vi "输入数据解析.vi"(0 "单个参数补充":dbl, 1 "从板号":dbl=1.0, 2 "主板二维码":string="BNET01", 3 "从板二维码":string="BNET01", 5 "主板引用":refnum<vi>, 7 "从板引用":refnum<vi>, 9 "主板选项":string="三级故障阀值", 11 "枚举":enum16{"主板", "从板"}(ring), 12 "快换":bool caption="快换写入") -> (4 "输出数组":dbl[][](array[numeric]), 6 "数组长度":dbl[](array[numeric]), 8 "循环次数":i32, 10 "命令":u32, 14 "名称":string[](array[string]), 15 "命令序号":u32[](array[numeric]))   [LabVIEW 2013] (continued)
          n2890 = Build Array(w7237) -> (w7236:dbl[][])
          n2891 = Build Array("一级故障阀值") -> (w7227:string[])
        }
        frame "充电电流过高(2)" {
          n2892 = Unbundle By Name(w7462) -> ("一级故障 2"=w7463:refnum<vi>)
          n2893 = property class="Clust (严格)"(reference=w7463) -> ("Value"=w7461:T4)  [unwired: 1 in, 2 out]
          n2894 = for {
            N: 17 -> [_]
            tunnel: w7461 -> [w7473]
            shift-right: [w7470] -> w7467
            shift-left: dbl[] [] -> [w7471]
            i -> [w7474]
            n2895 = case shown="13" w7474 {
              tunnel: w7473 -> [w7475 w7486 w7497 w7507 w7517 w7527 w7539 w7551 w7563 w7575 w7587 w7599 w7613 w7634 w7646 w7655 w7664]
              tunnel: [w7476 w7487 w7498 w7508 w7518 w7529 w7541 w7553 w7565 w7577 w7589 w7600 w7622 w7637 w7645 w7654 w7666] -> w7472
              frame 0, Default {
                # "总电压过高"
                n2896 = disable-structure shown="启用" {
                  disable-tunnel: [w7482 w7485] -> w7478
                  disable-tunnel: [w7481 w7485] -> w7477
                  disable-tunnel: w7475 -> [w7480 _]
                  frame Disabled {
                    n2897 = Unbundle By Name(w7480) -> ("总电压过高"=w7479:dbl)
                    n2898 = call "输入分辨率计算-EV05.vi"("1字节?"=FALSE, "数值"=w7479, "分辨率"=0.1) -> ("低字节"=w7482:dbl, "高字节1"=w7481:dbl)  [unwired: 2 in, 5 out]
                  }
                  frame Enabled {
                    w7485 = 255 ("高字节1")
                  }
                }
                n2899 = Build Array(w7477, w7478) -> (w7476:i32[])
              }
              frame 1 {
                # "总电压过低"
                n2900 = disable-structure shown="启用" {
                  disable-tunnel: [w7493 w7496] -> w7489
                  disable-tunnel: [w7492 w7496] -> w7488
                  disable-tunnel: w7486 -> [w7491 _]
                  frame Disabled {
                    n2901 = Unbundle By Name(w7491) -> ("总电压过低"=w7490:dbl)
                    n2902 = call "输入分辨率计算-EV05.vi"("1字节?"=FALSE, "数值"=w7490, "分辨率"=0.1) -> ("低字节"=w7493:dbl, "高字节1"=w7492:dbl)  [unwired: 2 in, 5 out]
                  }
                  frame Enabled {
                    w7496 = 255 ("高字节1")
                  }
                }
                n2903 = Build Array(w7488, w7489) -> (w7487:i32[])
              }
              frame 2 {
                # "温度过高"
                n2904 = disable-structure shown="启用" {
                  disable-tunnel: [w7503 255 ("高字节1")] -> w7499
                  disable-tunnel: w7497 -> [w7501 _]
                  frame Disabled {
                    n2905 = Unbundle By Name(w7501) -> ("温度过高"=w7500:dbl)
                    n2906 = call "输入分辨率计算-EV05.vi"("1字节?"=TRUE, "数值"=w7500, "偏移量"=-40.0, "分辨率"=1.0) -> ("高字节1"=w7503:dbl)  [unwired: 1 in, 6 out]
                  }
                  frame Enabled {
                  }
                }
                n2907 = Build Array(w7499) -> (w7498:i32[])
              }
              frame 3 {
                # "温度过低"
                n2908 = disable-structure shown="启用" {
                  disable-tunnel: [w7513 255 ("高字节1")] -> w7509
                  disable-tunnel: w7507 -> [w7511 _]
                  frame Disabled {
                    n2909 = Unbundle By Name(w7511) -> ("温度过低"=w7510:dbl)
                    n2910 = call "输入分辨率计算-EV05.vi"("1字节?"=TRUE, "数值"=w7510, "偏移量"=-40.0, "分辨率"=1.0) -> ("高字节1"=w7513:dbl)  [unwired: 1 in, 6 out]
                  }
                  frame Enabled {
                  }
                }
                n2911 = Build Array(w7509) -> (w7508:i32[])
              }
              frame 4 {
                # "整组温度不均衡"
                n2912 = disable-structure shown="启用" {
                  disable-tunnel: [w7523 255 ("高字节1")] -> w7519
                  disable-tunnel: w7517 -> [w7521 _]
                  frame Disabled {
                    n2913 = Unbundle By Name(w7521) -> ("整组温度不均衡"=w7520:dbl)
                    n2914 = call "输入分辨率计算-EV05.vi"("1字节?"=TRUE, "数值"=w7520, "偏移量"=0.0, "分辨率"=1.0) -> ("高字节1"=w7523:dbl)  [unwired: 1 in, 6 out]
                  }
                  frame Enabled {
                  }
                }
                n2915 = Build Array(w7519) -> (w7518:i32[])
              }
              frame 5 {
                # "单组电压不均衡"
                n2916 = disable-structure shown="启用" {
                  disable-tunnel: [w7535 w7538] -> w7530
                  disable-tunnel: [w7533 w7538] -> w7528
                  disable-tunnel: w7527 -> [w7532 _]
                  frame Disabled {
                    n2917 = Unbundle By Name(w7532) -> ("单组电压不均衡"=w7531:dbl)
                    n2918 = call "输入分辨率计算-EV05.vi"("1字节?"=FALSE, "数值"=w7531, "偏移量"=0.0, "分辨率"=0.001) -> ("低字节"=w7533:dbl, "高字节1"=w7535:dbl)  [unwired: 1 in, 5 out]
                  }
                  frame Enabled {
                    w7538 = 255 ("高字节1")
                  }
                }
                n2919 = Build Array(w7530, w7528) -> (w7529:i32[])
              }
              frame 6 {
                # "整组电压不均衡"
                n2920 = disable-structure shown="启用" {
                  disable-tunnel: [w7547 w7550] -> w7542
                  disable-tunnel: [w7545 w7550] -> w7540
                  disable-tunnel: w7539 -> [w7544 _]
                  frame Disabled {
                    n2921 = Unbundle By Name(w7544) -> ("整组电压不均衡"=w7543:dbl)
                    n2922 = call "输入分辨率计算-EV05.vi"("1字节?"=FALSE, "数值"=w7543, "偏移量"=0.0, "分辨率"=0.001) -> ("低字节"=w7545:dbl, "高字节1"=w7547:dbl)  [unwired: 1 in, 5 out]
                  }
                  frame Enabled {
                    w7550 = 255 ("高字节1")
                  }
                }
                n2923 = Build Array(w7542, w7540) -> (w7541:i32[])
              }
              frame 7 {
                # "单体电压过高"
                n2924 = disable-structure shown="启用" {
                  disable-tunnel: [w7559 w7562] -> w7554
                  disable-tunnel: [w7557 w7562] -> w7552
                  disable-tunnel: w7551 -> [w7556 _]
                  frame Disabled {
                    n2925 = Unbundle By Name(w7556) -> ("单体电压过高"=w7555:dbl)
                    n2926 = call "输入分辨率计算-EV05.vi"("1字节?"=FALSE, "数值"=w7555, "偏移量"=0.0, "分辨率"=0.001) -> ("低字节"=w7557:dbl, "高字节1"=w7559:dbl)  [unwired: 1 in, 5 out]
                  }
                  frame Enabled {
                    w7562 = 255 ("高字节1")
                  }
                }
                n2927 = Build Array(w7554, w7552) -> (w7553:i32[])
              }
              frame 8 {
                # "单体电压过低"
                n2928 = disable-structure shown="启用" {
                  disable-tunnel: [w7571 w7574] -> w7566
                  disable-tunnel: [w7569 w7574] -> w7564
                  disable-tunnel: w7563 -> [w7568 _]
                  frame Disabled {
                    n2929 = Unbundle By Name(w7568) -> ("单体电压过低"=w7567:dbl)
                    n2930 = call "输入分辨率计算-EV05.vi"("1字节?"=FALSE, "数值"=w7567, "偏移量"=0.0, "分辨率"=0.001) -> ("低字节"=w7569:dbl, "高字节1"=w7571:dbl)  [unwired: 1 in, 5 out]
                  }
                  frame Enabled {
                    w7574 = 255 ("高字节1")
                  }
                }
                n2931 = Build Array(w7566, w7564) -> (w7565:i32[])
              }
              frame 9 {
                # "充电电流过高"
                n2932 = disable-structure shown="启用" {
                  disable-tunnel: [w7583 w7586] -> w7578
                  disable-tunnel: [w7581 w7586] -> w7576
                  disable-tunnel: w7575 -> [w7580 _]
                  frame Enabled {
                    n2933 = Unbundle By Name(w7580) -> ("充电电流过高"=w7579:dbl)
                    n2934 = call "输入分辨率计算-EV05.vi"("1字节?"=FALSE, "数值"=w7579, "偏移量"=0.0, "分辨率"=0.1) -> ("低字节"=w7581:dbl, "高字节1"=w7583:dbl)  [unwired: 1 in, 5 out]
                  }
                  frame Disabled {
                    w7586 = 255 ("高字节1")
                  }
                }
                n2935 = Build Array(w7578, w7576) -> (w7577:dbl[])
              }
              frame 10 {
                # "放电电流过高"
                n2936 = disable-structure shown="启用" {
                  disable-tunnel: [w7595 w7598] -> w7590
                  disable-tunnel: [w7593 w7598] -> w7588
                  disable-tunnel: w7587 -> [w7592 _]
                  frame Disabled {
                    n2937 = Unbundle By Name(w7592) -> ("放电电流过高"=w7591:dbl)
                    n2938 = call "输入分辨率计算-EV05.vi"("1字节?"=FALSE, "数值"=w7591, "偏移量"=-3000.0, "分辨率"=0.1) -> ("低字节"=w7593:dbl, "高字节1"=w7595:dbl)  [unwired: 1 in, 5 out]
                  }
                  frame Enabled {
                    w7598 = 255 ("高字节1")
                  }
                }
                n2939 = Build Array(w7590, w7588) -> (w7589:i32[])
              }
              frame 11 {
                # "单组温度不均衡"
                n2940 = disable-structure shown="启用" {
                  disable-tunnel: [w7605 255 ("高字节1")] -> w7601
                  disable-tunnel: w7599 -> [w7603 _]
                  frame Disabled {
                    n2941 = Unbundle By Name(w7603) -> ("单组温度不均衡"=w7602:dbl)
                    n2942 = call "输入分辨率计算-EV05.vi"("1字节?"=TRUE, "数值"=w7602, "偏移量"=0.0, "分辨率"=1.0) -> ("高字节1"=w7605:dbl)  [unwired: 1 in, 6 out]
                  }
                  frame Enabled {
                  }
                }
                n2943 = Build Array(w7601) -> (w7600:i32[])
              }
              frame 12 {
                # "SOC过高"
                n2944 = Unbundle By Name(w7613) -> ("SOC过高"=w7612:dbl)
                n2945 = call "输入分辨率计算-EV05.vi"("1字节?"=FALSE, "数值"=w7612, "偏移量"=0.0, "分辨率"=0.1) -> ("低字节"=w7614:dbl, "高字节1"=w7615:dbl)  [unwired: 1 in, 5 out]
                n2946 = call "二进制解析-8.6.vi"("索引"=4, "数值"=w7615) -> ("低位子数组"=w7618:i32[])  [unwired: 3 out]
                n2947 = call "二进制解析-8.6.vi"("索引"=4, "数值"=w7614) -> ("低位子数组"=w7610:i32[], "高位子数组"=w7617:i32[])  [unwired: 2 out]
                n2948 = Insert Into Array(array=w7618, new element=w7617) -> (w7616:i32[])  [unwired: 1 in]
                n2949 = call "数值二进制转十进制-8.6.vi"("子数组"=w7616) -> ("十进制数值"=w7611:i32)  [unwired: 4 out]
                n2950 = disable-structure shown="启用" {
                  disable-tunnel: w7611 -> [w7626 _]
                  disable-tunnel: [w7626 255 ("高字节1")] -> w7609
                  disable-tunnel: [w7625 i32[] [] ("低位子数组 27")] -> _
                  disable-tunnel: w7610 -> [w7625 _]
                  frame Disabled {
                  }
                  frame Enabled {
                  }
                }
                n2951 = Build Array(w7609, w7609) -> (w7622:i32[])
              }
              frame 13 {
                # "SOC过低"
                n2952 = Unbundle By Name(w7634) -> ("SOC过低"=w7633:dbl)
                n2953 = call "输入分辨率计算-EV05.vi"("1字节?"=FALSE, "数值"=w7633, "偏移量"=0.0, "分辨率"=0.1) -> ("低字节"=w7631:dbl, "高字节1"=w7632:dbl)  [unwired: 1 in, 5 out]
                n2954 = call "二进制解析-8.6.vi"("索引"=4, "数值"=w7632) -> ("低位子数组"=w7630:i32[])  [unwired: 3 out]
                n2955 = disable-structure shown="启用" {
                  disable-tunnel: w7631 -> [w7641 _]
                  disable-tunnel: [w7641 255 ("高字节1")] -> w7629
                  disable-tunnel: w7630 -> [w7640 _]
                  disable-tunnel: [w7640 i32[] [] ("低位子数组")] -> _
                  frame Disabled {
                    (unwired) i32[] [] ("低位子数组 4")
                  }
                  frame Enabled {
                  }
                }
                n2956 = Build Array(w7629, w7629) -> (w7637:i32[])
              }
              frame 14 {
                # "内阻过大"
                n2957 = disable-structure shown="启用" {
                  disable-tunnel: w7646 -> [w7651 _]
                  disable-tunnel: [w7647 255 ("高字节1")] -> w7644
                  frame Disabled {
                    n2958 = Unbundle By Name(w7651) -> ("内阻过大"=w7650:dbl)
                    n2959 = call "输入分辨率计算-EV05.vi"("1字节?"=TRUE, "数值"=w7650, "分辨率"=0.1) -> ("高字节1"=w7647:dbl)  [unwired: 2 in, 6 out]
                  }
                  frame Enabled {
                  }
                }
                n2960 = Build Array(w7644) -> (w7645:i32[])
              }
              frame 15 {
                # "极柱温度过高"
                n2961 = disable-structure shown="启用" {
                  disable-tunnel: w7655 -> [w7661 _]
                  disable-tunnel: [w7657 255 ("高字节1")] -> w7653
                  frame Disabled {
                    n2962 = Unbundle By Name(w7661) -> ("极柱温度过高"=w7660:dbl)
                    n2963 = call "输入分辨率计算-EV05.vi"("1字节?"=TRUE, "数值"=w7660, "偏移量"=-40.0, "分辨率"=1.0) -> ("高字节1"=w7657:dbl)  [unwired: 1 in, 6 out]
                  }
                  frame Enabled {
                  }
                }
                n2964 = Build Array(w7653) -> (w7654:i32[])
              }
              frame 16 {
                # "SOH过低"
                n2965 = disable-structure shown="启用" {
                  disable-tunnel: [w7678 w7686] -> w7665
                  disable-tunnel: w7664 -> [w7675 _]
                  disable-tunnel: [w7667 w7686] -> w7663
                  frame Disabled {
                    n2966 = Unbundle By Name(w7675) -> ("SOH过低"=w7674:dbl)
                    n2967 = call "输入分辨率计算-EV05.vi"("1字节?"=FALSE, "数值"=w7674, "偏移量"=0.0, "分辨率"=0.1) -> ("低字节"=w7676:dbl, "高字节1"=w7677:dbl)  [unwired: 1 in, 5 out]
                    n2968 = call "二进制解析-8.6.vi"("索引"=4, "数值"=w7677) -> ("低位子数组"=w7680:i32[])  [unwired: 3 out]
                    n2969 = call "二进制解析-8.6.vi"("索引"=4, "数值"=w7676) -> ("低位子数组"=w7669:i32[], "高位子数组"=w7679:i32[])  [unwired: 2 out]
                    n2970 = call "二进制解析-8.6.vi"("索引"=4, "数值"=0) -> ("低位子数组"=w7670:i32[])  [unwired: 3 out]
                    n2971 = Insert Into Array(array=w7680, new element=w7679) -> (w7673:i32[])  [unwired: 1 in]
                    n2972 = Insert Into Array(array=w7669, new element=w7670) -> (w7668:i32[])  [unwired: 1 in]
                    n2973 = call "数值二进制转十进制-8.6.vi"("子数组"=w7673) -> ("十进制数值"=w7678:i32)  [unwired: 4 out]
                    n2974 = call "数值二进制转十进制-8.6.vi"("子数组"=w7668) -> ("十进制数值"=w7667:i32)  [unwired: 4 out]
                  }
                  frame Enabled {
                    w7686 = 255 ("高字节1")
                  }
                }
                n2975 = Build Array(w7665, w7663) -> (w7666:i32[])
              }
            }
            n2976 = Insert Into Array(array=w7471, new element=w7472) -> (w7470:dbl[])  [unwired: 1 in]
          }
          n2977 = Build Array(w7467) -> (w7466:dbl[][])
          n2978 = Build Array("二级故障阀值") -> (w7457:string[])
        }
        frame "充电电流过高(3)" {
          n2979 = Unbundle By Name(w7692) -> ("一级故障 3"=w7693:refnum<vi>)
          n2980 = property class="Clust (严格)"(reference=w7693) -> ("Value"=w7691:T4)  [unwired: 1 in, 2 out]
          n2981 = for {
            N: 17 -> [_]
            tunnel: w7691 -> [w7703]
            shift-right: [w7700] -> w7697
            shift-left: dbl[] [] -> [w7701]
            i -> [w7704]
            n2982 = case shown="13" w7704 {
              tunnel: w7703 -> [w7705 w7716 w7727 w7737 w7747 w7757 w7769 w7781 w7793 w7805 w7817 w7829 w7843 w7864 w7876 w7885 w7894]
              tunnel: [w7706 w7717 w7728 w7738 w7748 w7759 w7771 w7783 w7795 w7807 w7819 w7830 w7852 w7867 w7875 w7884 w7896] -> w7702
              frame 0, Default {
                # "总电压过高"
                n2983 = disable-structure shown="启用" {
                  disable-tunnel: [w7712 w7715] -> w7708
                  disable-tunnel: [w7711 w7715] -> w7707
                  disable-tunnel: w7705 -> [w7710 _]
                  frame Disabled {
                    n2984 = Unbundle By Name(w7710) -> ("总电压过高"=w7709:dbl)
                    n2985 = call "输入分辨率计算-EV05.vi"("1字节?"=FALSE, "数值"=w7709, "分辨率"=0.1) -> ("低字节"=w7712:dbl, "高字节1"=w7711:dbl)  [unwired: 2 in, 5 out]
                  }
                  frame Enabled {
                    w7715 = 255 ("高字节1")
                  }
                }
                n2986 = Build Array(w7707, w7708) -> (w7706:i32[])
              }
              frame 1 {
                # "总电压过低"
                n2987 = disable-structure shown="启用" {
                  disable-tunnel: [w7723 w7726] -> w7719
                  disable-tunnel: [w7722 w7726] -> w7718
                  disable-tunnel: w7716 -> [w7721 _]
                  frame Disabled {
                    n2988 = Unbundle By Name(w7721) -> ("总电压过低"=w7720:dbl)
                    n2989 = call "输入分辨率计算-EV05.vi"("1字节?"=FALSE, "数值"=w7720, "分辨率"=0.1) -> ("低字节"=w7723:dbl, "高字节1"=w7722:dbl)  [unwired: 2 in, 5 out]
                  }
                  frame Enabled {
                    w7726 = 255 ("高字节1")
                  }
                }
                n2990 = Build Array(w7718, w7719) -> (w7717:i32[])
              }
              frame 2 {
                # "温度过高"
                n2991 = disable-structure shown="启用" {
                  disable-tunnel: [w7733 255 ("高字节1")] -> w7729
                  disable-tunnel: w7727 -> [w7731 _]
                  frame Disabled {
                    n2992 = Unbundle By Name(w7731) -> ("温度过高"=w7730:dbl)
                    n2993 = call "输入分辨率计算-EV05.vi"("1字节?"=TRUE, "数值"=w7730, "偏移量"=-40.0, "分辨率"=1.0) -> ("高字节1"=w7733:dbl)  [unwired: 1 in, 6 out]
                  }
                  frame Enabled {
                  }
                }
                n2994 = Build Array(w7729) -> (w7728:i32[])
              }
              frame 3 {
                # "温度过低"
                n2995 = disable-structure shown="启用" {
                  disable-tunnel: [w7743 255 ("高字节1")] -> w7739
                  disable-tunnel: w7737 -> [w7741 _]
                  frame Disabled {
                    n2996 = Unbundle By Name(w7741) -> ("温度过低"=w7740:dbl)
                    n2997 = call "输入分辨率计算-EV05.vi"("1字节?"=TRUE, "数值"=w7740, "偏移量"=-40.0, "分辨率"=1.0) -> ("高字节1"=w7743:dbl)  [unwired: 1 in, 6 out]
                  }
                  frame Enabled {
                  }
                }
                n2998 = Build Array(w7739) -> (w7738:i32[])
              }
              frame 4 {
                # "整组温度不均衡"
                n2999 = disable-structure shown="启用" {
                  disable-tunnel: [w7753 255 ("高字节1")] -> w7749
                  disable-tunnel: w7747 -> [w7751 _]
                  frame Disabled {
                    n3000 = Unbundle By Name(w7751) -> ("整组温度不均衡"=w7750:dbl)
                    n3001 = call "输入分辨率计算-EV05.vi"("1字节?"=TRUE, "数值"=w7750, "偏移量"=0.0, "分辨率"=1.0) -> ("高字节1"=w7753:dbl)  [unwired: 1 in, 6 out]
                  }
                  frame Enabled {
                  }
                }
                n3002 = Build Array(w7749) -> (w7748:i32[])
              }
              frame 5 {
                # "单组电压不均衡"
                n3003 = disable-structure shown="启用" {
                  disable-tunnel: [w7765 w7768] -> w7760
                  disable-tunnel: [w7763 w7768] -> w7758
                  disable-tunnel: w7757 -> [w7762 _]
                  frame Disabled {
                    n3004 = Unbundle By Name(w7762) -> ("单组电压不均衡"=w7761:dbl)
                    n3005 = call "输入分辨率计算-EV05.vi"("1字节?"=FALSE, "数值"=w7761, "偏移量"=0.0, "分辨率"=0.001) -> ("低字节"=w7763:dbl, "高字节1"=w7765:dbl)  [unwired: 1 in, 5 out]
                  }
                  frame Enabled {
                    w7768 = 255 ("高字节1")
                  }
                }
                n3006 = Build Array(w7760, w7758) -> (w7759:i32[])
              }
              frame 6 {
                # "整组电压不均衡"
                n3007 = disable-structure shown="启用" {
                  disable-tunnel: [w7777 w7780] -> w7772
                  disable-tunnel: [w7775 w7780] -> w7770
                  disable-tunnel: w7769 -> [w7774 _]
                  frame Disabled {
                    n3008 = Unbundle By Name(w7774) -> ("整组电压不均衡"=w7773:dbl)
                    n3009 = call "输入分辨率计算-EV05.vi"("1字节?"=FALSE, "数值"=w7773, "偏移量"=0.0, "分辨率"=0.001) -> ("低字节"=w7775:dbl, "高字节1"=w7777:dbl)  [unwired: 1 in, 5 out]
                  }
                  frame Enabled {
                    w7780 = 255 ("高字节1")
                  }
                }
                n3010 = Build Array(w7772, w7770) -> (w7771:i32[])
              }
              frame 7 {
                # "单体电压过高"
                n3011 = disable-structure shown="启用" {
                  disable-tunnel: [w7789 w7792] -> w7784
                  disable-tunnel: [w7787 w7792] -> w7782
                  disable-tunnel: w7781 -> [w7786 _]
                  frame Disabled {
                    n3012 = Unbundle By Name(w7786) -> ("单体电压过高"=w7785:dbl)
                    n3013 = call "输入分辨率计算-EV05.vi"("1字节?"=FALSE, "数值"=w7785, "偏移量"=0.0, "分辨率"=0.001) -> ("低字节"=w7787:dbl, "高字节1"=w7789:dbl)  [unwired: 1 in, 5 out]
                  }
                  frame Enabled {
                    w7792 = 255 ("高字节1")
                  }
                }
                n3014 = Build Array(w7784, w7782) -> (w7783:i32[])
              }
              frame 8 {
                # "单体电压过低"
                n3015 = disable-structure shown="启用" {
                  disable-tunnel: [w7801 w7804] -> w7796
                  disable-tunnel: [w7799 w7804] -> w7794
                  disable-tunnel: w7793 -> [w7798 _]
                  frame Disabled {
                    n3016 = Unbundle By Name(w7798) -> ("单体电压过低"=w7797:dbl)
                    n3017 = call "输入分辨率计算-EV05.vi"("1字节?"=FALSE, "数值"=w7797, "偏移量"=0.0, "分辨率"=0.001) -> ("低字节"=w7799:dbl, "高字节1"=w7801:dbl)  [unwired: 1 in, 5 out]
                  }
                  frame Enabled {
                    w7804 = 255 ("高字节1")
                  }
                }
                n3018 = Build Array(w7796, w7794) -> (w7795:i32[])
              }
              frame 9 {
                # "充电电流过高"
                n3019 = disable-structure shown="启用" {
                  disable-tunnel: [w7813 w7816] -> w7808
                  disable-tunnel: [w7811 w7816] -> w7806
                  disable-tunnel: w7805 -> [w7810 _]
                  frame Enabled {
                    n3020 = Unbundle By Name(w7810) -> ("充电电流过高"=w7809:dbl)
                    n3021 = call "输入分辨率计算-EV05.vi"("1字节?"=FALSE, "数值"=w7809, "偏移量"=0.0, "分辨率"=0.1) -> ("低字节"=w7811:dbl, "高字节1"=w7813:dbl)  [unwired: 1 in, 5 out]
                  }
                  frame Disabled {
                    w7816 = 255 ("高字节1")
                  }
                }
                n3022 = Build Array(w7808, w7806) -> (w7807:dbl[])
              }
              frame 10 {
                # "放电电流过高"
                n3023 = disable-structure shown="启用" {
                  disable-tunnel: [w7825 w7828] -> w7820
                  disable-tunnel: [w7823 w7828] -> w7818
                  disable-tunnel: w7817 -> [w7822 _]
                  frame Disabled {
                    n3024 = Unbundle By Name(w7822) -> ("放电电流过高"=w7821:dbl)
                    n3025 = call "输入分辨率计算-EV05.vi"("1字节?"=FALSE, "数值"=w7821, "偏移量"=-3000.0, "分辨率"=0.1) -> ("低字节"=w7823:dbl, "高字节1"=w7825:dbl)  [unwired: 1 in, 5 out]
                  }
                  frame Enabled {
                    w7828 = 255 ("高字节1")
                  }
                }
                n3026 = Build Array(w7820, w7818) -> (w7819:i32[])
              }
              frame 11 {
                # "单组温度不均衡"
                n3027 = disable-structure shown="启用" {
                  disable-tunnel: [w7835 255 ("高字节1")] -> w7831
                  disable-tunnel: w7829 -> [w7833 _]
                  frame Disabled {
                    n3028 = Unbundle By Name(w7833) -> ("单组温度不均衡"=w7832:dbl)
                    n3029 = call "输入分辨率计算-EV05.vi"("1字节?"=TRUE, "数值"=w7832, "偏移量"=0.0, "分辨率"=1.0) -> ("高字节1"=w7835:dbl)  [unwired: 1 in, 6 out]
                  }
                  frame Enabled {
                  }
                }
                n3030 = Build Array(w7831) -> (w7830:i32[])
              }
              frame 12 {
                # "SOC过高"
                n3031 = Unbundle By Name(w7843) -> ("SOC过高"=w7842:dbl)
                n3032 = call "输入分辨率计算-EV05.vi"("1字节?"=FALSE, "数值"=w7842, "偏移量"=0.0, "分辨率"=0.1) -> ("低字节"=w7844:dbl, "高字节1"=w7845:dbl)  [unwired: 1 in, 5 out]
                n3033 = call "二进制解析-8.6.vi"("索引"=4, "数值"=w7845) -> ("低位子数组"=w7848:i32[])  [unwired: 3 out]
                n3034 = call "二进制解析-8.6.vi"("索引"=4, "数值"=w7844) -> ("低位子数组"=w7840:i32[], "高位子数组"=w7847:i32[])  [unwired: 2 out]
                n3035 = Insert Into Array(array=w7848, new element=w7847) -> (w7846:i32[])  [unwired: 1 in]
                n3036 = call "数值二进制转十进制-8.6.vi"("子数组"=w7846) -> ("十进制数值"=w7841:i32)  [unwired: 4 out]
                n3037 = disable-structure shown="启用" {
                  disable-tunnel: w7841 -> [w7856 _]
                  disable-tunnel: [w7856 255 ("高字节1")] -> w7839
                  disable-tunnel: [w7855 i32[] [] ("低位子数组 27")] -> _
                  disable-tunnel: w7840 -> [w7855 _]
                  frame Disabled {
                  }
                  frame Enabled {
                  }
                }
                n3038 = Build Array(w7839, w7839) -> (w7852:i32[])
              }
              frame 13 {
                # "SOC过低"
                n3039 = Unbundle By Name(w7864) -> ("SOC过低"=w7863:dbl)
                n3040 = call "输入分辨率计算-EV05.vi"("1字节?"=FALSE, "数值"=w7863, "偏移量"=0.0, "分辨率"=0.1) -> ("低字节"=w7861:dbl, "高字节1"=w7862:dbl)  [unwired: 1 in, 5 out]
                n3041 = call "二进制解析-8.6.vi"("索引"=4, "数值"=w7862) -> ("低位子数组"=w7860:i32[])  [unwired: 3 out]
                n3042 = disable-structure shown="启用" {
                  disable-tunnel: w7861 -> [w7871 _]
                  disable-tunnel: [w7871 255 ("高字节1")] -> w7859
                  disable-tunnel: w7860 -> [w7870 _]
                  disable-tunnel: [w7870 i32[] [] ("低位子数组")] -> _
                  frame Disabled {
                    (unwired) i32[] [] ("低位子数组 4")
                  }
                  frame Enabled {
                  }
                }
                n3043 = Build Array(w7859, w7859) -> (w7867:i32[])
              }
              frame 14 {
                # "内阻过大"
                n3044 = disable-structure shown="启用" {
                  disable-tunnel: w7876 -> [w7881 _]
                  disable-tunnel: [w7877 255 ("高字节1")] -> w7874
                  frame Disabled {
                    n3045 = Unbundle By Name(w7881) -> ("内阻过大"=w7880:dbl)
                    n3046 = call "输入分辨率计算-EV05.vi"("1字节?"=TRUE, "数值"=w7880, "分辨率"=0.1) -> ("高字节1"=w7877:dbl)  [unwired: 2 in, 6 out]
                  }
                  frame Enabled {
                  }
                }
                n3047 = Build Array(w7874) -> (w7875:i32[])
              }
              frame 15 {
                # "极柱温度过高"
                n3048 = disable-structure shown="启用" {
                  disable-tunnel: w7885 -> [w7891 _]
                  disable-tunnel: [w7887 255 ("高字节1")] -> w7883
                  frame Disabled {
                    n3049 = Unbundle By Name(w7891) -> ("极柱温度过高"=w7890:dbl)
                    n3050 = call "输入分辨率计算-EV05.vi"("1字节?"=TRUE, "数值"=w7890, "偏移量"=-40.0, "分辨率"=1.0) -> ("高字节1"=w7887:dbl)  [unwired: 1 in, 6 out]
                  }
                  frame Enabled {
                  }
                }
                n3051 = Build Array(w7883) -> (w7884:i32[])
              }
              frame 16 {
                # "SOH过低"
                n3052 = disable-structure shown="启用" {
                  disable-tunnel: [w7908 w7916] -> w7895
                  disable-tunnel: w7894 -> [w7905 _]
                  disable-tunnel: [w7897 w7916] -> w7893
                  frame Disabled {
                    n3053 = Unbundle By Name(w7905) -> ("SOH过低"=w7904:dbl)
                    n3054 = call "输入分辨率计算-EV05.vi"("1字节?"=FALSE, "数值"=w7904, "偏移量"=0.0, "分辨率"=0.1) -> ("低字节"=w7906:dbl, "高字节1"=w7907:dbl)  [unwired: 1 in, 5 out]
                    n3055 = call "二进制解析-8.6.vi"("索引"=4, "数值"=w7907) -> ("低位子数组"=w7910:i32[])  [unwired: 3 out]
                    n3056 = call "二进制解析-8.6.vi"("索引"=4, "数值"=w7906) -> ("低位子数组"=w7899:i32[], "高位子数组"=w7909:i32[])  [unwired: 2 out]
                    n3057 = call "二进制解析-8.6.vi"("索引"=4, "数值"=0) -> ("低位子数组"=w7900:i32[])  [unwired: 3 out]
                    n3058 = Insert Into Array(array=w7910, new element=w7909) -> (w7903:i32[])  [unwired: 1 in]
                    n3059 = Insert Into Array(array=w7899, new element=w7900) -> (w7898:i32[])  [unwired: 1 in]
                    n3060 = call "数值二进制转十进制-8.6.vi"("子数组"=w7903) -> ("十进制数值"=w7908:i32)  [unwired: 4 out]
                    n3061 = call "数值二进制转十进制-8.6.vi"("子数组"=w7898) -> ("十进制数值"=w7897:i32)  [unwired: 4 out]
                  }
                  frame Enabled {
                    w7916 = 255 ("高字节1")
                  }
                }
                n3062 = Build Array(w7895, w7893) -> (w7896:i32[])
              }
            }
            n3063 = Insert Into Array(array=w7701, new element=w7702) -> (w7700:dbl[])  [unwired: 1 in]
          }
          n3064 = Build Array(w7697) -> (w7696:dbl[][])
          n3065 = Build Array("三级故障阀值") -> (w7687:string[])
        }
        frame "放电电流过高" {
          n3066 = Unbundle By Name(w7922) -> ("一级故障"=w7923:refnum<vi>)
          n3067 = property class="Clust (严格)"(reference=w7923) -> ("Value"=w7921:T4)  [unwired: 1 in, 2 out]
          n3068 = for {
            N: 17 -> [_]
            tunnel: w7921 -> [w7933]
            shift-right: [w7930] -> w7927
            shift-left: dbl[] [] -> [w7931]
            i -> [w7934]
            n3069 = case shown="14" w7934 {
              tunnel: w7933 -> [w7935 w7946 w7957 w7967 w7977 w7987 w7999 w8011 w8023 w8035 w8047 w8059 w8073 w8094 w8106 w8115 w8124]
              tunnel: [w7936 w7947 w7958 w7968 w7978 w7989 w8001 w8013 w8025 w8037 w8049 w8060 w8082 w8097 w8105 w8114 w8126] -> w7932
              frame 0, Default {
                # "总电压过高"
                n3070 = disable-structure shown="启用" {
                  disable-tunnel: [w7942 w7945] -> w7938
                  disable-tunnel: [w7941 w7945] -> w7937
                  disable-tunnel: w7935 -> [w7940 _]
                  frame Disabled {
                    n3071 = Unbundle By Name(w7940) -> ("总电压过高"=w7939:dbl)
                    n3072 = call "输入分辨率计算-EV05.vi"("1字节?"=FALSE, "数值"=w7939, "分辨率"=0.1) -> ("低字节"=w7942:dbl, "高字节1"=w7941:dbl)  [unwired: 2 in, 5 out]
                  }
                  frame Enabled {
                    w7945 = 255 ("高字节1")
                  }
                }
                n3073 = Build Array(w7937, w7938) -> (w7936:i32[])
              }
              frame 1 {
                # "总电压过低"
                n3074 = disable-structure shown="启用" {
                  disable-tunnel: [w7953 w7956] -> w7949
                  disable-tunnel: [w7952 w7956] -> w7948
                  disable-tunnel: w7946 -> [w7951 _]
                  frame Disabled {
                    n3075 = Unbundle By Name(w7951) -> ("总电压过低"=w7950:dbl)
                    n3076 = call "输入分辨率计算-EV05.vi"("1字节?"=FALSE, "数值"=w7950, "分辨率"=0.1) -> ("低字节"=w7953:dbl, "高字节1"=w7952:dbl)  [unwired: 2 in, 5 out]
                  }
                  frame Enabled {
                    w7956 = 255 ("高字节1")
                  }
                }
                n3077 = Build Array(w7948, w7949) -> (w7947:i32[])
              }
              frame 2 {
                # "温度过高"
                n3078 = disable-structure shown="启用" {
                  disable-tunnel: [w7963 255 ("高字节1")] -> w7959
                  disable-tunnel: w7957 -> [w7961 _]
                  frame Disabled {
                    n3079 = Unbundle By Name(w7961) -> ("温度过高"=w7960:dbl)
                    n3080 = call "输入分辨率计算-EV05.vi"("1字节?"=TRUE, "数值"=w7960, "偏移量"=-40.0, "分辨率"=1.0) -> ("高字节1"=w7963:dbl)  [unwired: 1 in, 6 out]
                  }
                  frame Enabled {
                  }
                }
                n3081 = Build Array(w7959) -> (w7958:i32[])
              }
              frame 3 {
                # "温度过低"
                n3082 = disable-structure shown="启用" {
                  disable-tunnel: [w7973 255 ("高字节1")] -> w7969
                  disable-tunnel: w7967 -> [w7971 _]
                  frame Disabled {
                    n3083 = Unbundle By Name(w7971) -> ("温度过低"=w7970:dbl)
                    n3084 = call "输入分辨率计算-EV05.vi"("1字节?"=TRUE, "数值"=w7970, "偏移量"=-40.0, "分辨率"=1.0) -> ("高字节1"=w7973:dbl)  [unwired: 1 in, 6 out]
                  }
                  frame Enabled {
                  }
                }
                n3085 = Build Array(w7969) -> (w7968:i32[])
              }
              frame 4 {
                # "整组温度不均衡"
                n3086 = disable-structure shown="启用" {
                  disable-tunnel: [w7983 255 ("高字节1")] -> w7979
                  disable-tunnel: w7977 -> [w7981 _]
                  frame Disabled {
                    n3087 = Unbundle By Name(w7981) -> ("整组温度不均衡"=w7980:dbl)
                    n3088 = call "输入分辨率计算-EV05.vi"("1字节?"=TRUE, "数值"=w7980, "偏移量"=0.0, "分辨率"=1.0) -> ("高字节1"=w7983:dbl)  [unwired: 1 in, 6 out]
                  }
                  frame Enabled {
                  }
                }
                n3089 = Build Array(w7979) -> (w7978:i32[])
              }
              frame 5 {
                # "单组电压不均衡"
                n3090 = disable-structure shown="启用" {
                  disable-tunnel: [w7995 w7998] -> w7990
                  disable-tunnel: [w7993 w7998] -> w7988
                  disable-tunnel: w7987 -> [w7992 _]
                  frame Disabled {
                    n3091 = Unbundle By Name(w7992) -> ("单组电压不均衡"=w7991:dbl)
                    n3092 = call "输入分辨率计算-EV05.vi"("1字节?"=FALSE, "数值"=w7991, "偏移量"=0.0, "分辨率"=0.001) -> ("低字节"=w7993:dbl, "高字节1"=w7995:dbl)  [unwired: 1 in, 5 out]
                  }
                  frame Enabled {
                    w7998 = 255 ("高字节1")
                  }
                }
                n3093 = Build Array(w7990, w7988) -> (w7989:i32[])
              }
              frame 6 {
                # "整组电压不均衡"
                n3094 = disable-structure shown="启用" {
                  disable-tunnel: [w8007 w8010] -> w8002
                  disable-tunnel: [w8005 w8010] -> w8000
                  disable-tunnel: w7999 -> [w8004 _]
                  frame Disabled {
                    n3095 = Unbundle By Name(w8004) -> ("整组电压不均衡"=w8003:dbl)
                    n3096 = call "输入分辨率计算-EV05.vi"("1字节?"=FALSE, "数值"=w8003, "偏移量"=0.0, "分辨率"=0.001) -> ("低字节"=w8005:dbl, "高字节1"=w8007:dbl)  [unwired: 1 in, 5 out]
                  }
                  frame Enabled {
                    w8010 = 255 ("高字节1")
                  }
                }
                n3097 = Build Array(w8002, w8000) -> (w8001:i32[])
              }
              frame 7 {
                # "单体电压过高"
                n3098 = disable-structure shown="启用" {
                  disable-tunnel: [w8019 w8022] -> w8014
                  disable-tunnel: [w8017 w8022] -> w8012
                  disable-tunnel: w8011 -> [w8016 _]
                  frame Disabled {
                    n3099 = Unbundle By Name(w8016) -> ("单体电压过高"=w8015:dbl)
                    n3100 = call "输入分辨率计算-EV05.vi"("1字节?"=FALSE, "数值"=w8015, "偏移量"=0.0, "分辨率"=0.001) -> ("低字节"=w8017:dbl, "高字节1"=w8019:dbl)  [unwired: 1 in, 5 out]
                  }
                  frame Enabled {
                    w8022 = 255 ("高字节1")
                  }
                }
                n3101 = Build Array(w8014, w8012) -> (w8013:i32[])
              }
              frame 8 {
                # "单体电压过低"
                n3102 = disable-structure shown="启用" {
                  disable-tunnel: [w8031 w8034] -> w8026
                  disable-tunnel: [w8029 w8034] -> w8024
                  disable-tunnel: w8023 -> [w8028 _]
                  frame Disabled {
                    n3103 = Unbundle By Name(w8028) -> ("单体电压过低"=w8027:dbl)
                    n3104 = call "输入分辨率计算-EV05.vi"("1字节?"=FALSE, "数值"=w8027, "偏移量"=0.0, "分辨率"=0.001) -> ("低字节"=w8029:dbl, "高字节1"=w8031:dbl)  [unwired: 1 in, 5 out]
                  }
                  frame Enabled {
                    w8034 = 255 ("高字节1")
                  }
                }
                n3105 = Build Array(w8026, w8024) -> (w8025:i32[])
              }
              frame 9 {
                # "充电电流过高"
                n3106 = disable-structure shown="启用" {
                  disable-tunnel: [w8043 w8046] -> w8038
                  disable-tunnel: [w8041 w8046] -> w8036
                  disable-tunnel: w8035 -> [w8040 _]
                  frame Disabled {
                    n3107 = Unbundle By Name(w8040) -> ("充电电流过高"=w8039:dbl)
                    n3108 = call "输入分辨率计算-EV05.vi"("1字节?"=FALSE, "数值"=w8039, "偏移量"=-3000.0, "分辨率"=0.1) -> ("低字节"=w8041:dbl, "高字节1"=w8043:dbl)  [unwired: 1 in, 5 out]
                  }
                  frame Enabled {
                    w8046 = 255 ("高字节1")
                  }
                }
                n3109 = Build Array(w8038, w8036) -> (w8037:i32[])
              }
              frame 10 {
                # "放电电流过高"
                n3110 = disable-structure shown="启用" {
                  disable-tunnel: [w8055 w8058] -> w8050
                  disable-tunnel: [w8053 w8058] -> w8048
                  disable-tunnel: w8047 -> [w8052 _]
                  frame Enabled {
                    n3111 = Unbundle By Name(w8052) -> ("放电电流过高"=w8051:dbl)
                    n3112 = call "输入分辨率计算-EV05.vi"("1字节?"=FALSE, "数值"=w8051, "偏移量"=0.0, "分辨率"=0.1) -> ("低字节"=w8053:dbl, "高字节1"=w8055:dbl)  [unwired: 1 in, 5 out]
                  }
                  frame Disabled {
                    w8058 = 255 ("高字节1")
                  }
                }
                n3113 = Build Array(w8050, w8048) -> (w8049:dbl[])
              }
              frame 11 {
                # "单组温度不均衡"
                n3114 = disable-structure shown="启用" {
                  disable-tunnel: [w8065 255 ("高字节1")] -> w8061
                  disable-tunnel: w8059 -> [w8063 _]
                  frame Disabled {
                    n3115 = Unbundle By Name(w8063) -> ("单组温度不均衡"=w8062:dbl)
                    n3116 = call "输入分辨率计算-EV05.vi"("1字节?"=TRUE, "数值"=w8062, "偏移量"=0.0, "分辨率"=1.0) -> ("高字节1"=w8065:dbl)  [unwired: 1 in, 6 out]
                  }
                  frame Enabled {
                  }
                }
                n3117 = Build Array(w8061) -> (w8060:i32[])
              }
              frame 12 {
                # "SOC过高"
                n3118 = Unbundle By Name(w8073) -> ("SOC过高"=w8072:dbl)
                n3119 = call "输入分辨率计算-EV05.vi"("1字节?"=FALSE, "数值"=w8072, "偏移量"=0.0, "分辨率"=0.1) -> ("低字节"=w8074:dbl, "高字节1"=w8075:dbl)  [unwired: 1 in, 5 out]
                n3120 = call "二进制解析-8.6.vi"("索引"=4, "数值"=w8075) -> ("低位子数组"=w8078:i32[])  [unwired: 3 out]
                n3121 = call "二进制解析-8.6.vi"("索引"=4, "数值"=w8074) -> ("低位子数组"=w8070:i32[], "高位子数组"=w8077:i32[])  [unwired: 2 out]
                n3122 = Insert Into Array(array=w8078, new element=w8077) -> (w8076:i32[])  [unwired: 1 in]
                n3123 = call "数值二进制转十进制-8.6.vi"("子数组"=w8076) -> ("十进制数值"=w8071:i32)  [unwired: 4 out]
                n3124 = disable-structure shown="启用" {
                  disable-tunnel: w8071 -> [w8086 _]
                  disable-tunnel: [w8086 255 ("高字节1")] -> w8069
                  disable-tunnel: [w8085 i32[] [] ("低位子数组 28")] -> _
                  disable-tunnel: w8070 -> [w8085 _]
                  frame Disabled {
                  }
                  frame Enabled {
                  }
                }
                n3125 = Build Array(w8069, w8069) -> (w8082:i32[])
              }
              frame 13 {
                # "SOC过低"
                n3126 = Unbundle By Name(w8094) -> ("SOC过低"=w8093:dbl)
                n3127 = call "输入分辨率计算-EV05.vi"("1字节?"=FALSE, "数值"=w8093, "偏移量"=0.0, "分辨率"=0.1) -> ("低字节"=w8091:dbl, "高字节1"=w8092:dbl)  [unwired: 1 in, 5 out]
                n3128 = call "二进制解析-8.6.vi"("索引"=4, "数值"=w8092) -> ("低位子数组"=w8090:i32[])  [unwired: 3 out]
                n3129 = disable-structure shown="启用" {
                  disable-tunnel: w8091 -> [w8101 _]
                  disable-tunnel: [w8101 255 ("高字节1")] -> w8089
                  disable-tunnel: w8090 -> [w8100 _]
                  disable-tunnel: [w8100 i32[] [] ("低位子数组")] -> _
                  frame Disabled {
                    (unwired) i32[] [] ("低位子数组 4")
                  }
                  frame Enabled {
                  }
                }
                n3130 = Build Array(w8089, w8089) -> (w8097:i32[])
              }
              frame 14 {
                # "内阻过大"
                n3131 = disable-structure shown="启用" {
                  disable-tunnel: w8106 -> [w8111 _]
                  disable-tunnel: [w8107 255 ("高字节1")] -> w8104
                  frame Disabled {
                    n3132 = Unbundle By Name(w8111) -> ("内阻过大"=w8110:dbl)
                    n3133 = call "输入分辨率计算-EV05.vi"("1字节?"=TRUE, "数值"=w8110, "分辨率"=0.1) -> ("高字节1"=w8107:dbl)  [unwired: 2 in, 6 out]
                  }
                  frame Enabled {
                  }
                }
                n3134 = Build Array(w8104) -> (w8105:i32[])
              }
              frame 15 {
                # "极柱温度过高"
                n3135 = disable-structure shown="启用" {
                  disable-tunnel: w8115 -> [w8121 _]
                  disable-tunnel: [w8117 255 ("高字节1")] -> w8113
                  frame Disabled {
                    n3136 = Unbundle By Name(w8121) -> ("极柱温度过高"=w8120:dbl)
                    n3137 = call "输入分辨率计算-EV05.vi"("1字节?"=TRUE, "数值"=w8120, "偏移量"=-40.0, "分辨率"=1.0) -> ("高字节1"=w8117:dbl)  [unwired: 1 in, 6 out]
                  }
                  frame Enabled {
                  }
                }
                n3138 = Build Array(w8113) -> (w8114:i32[])
              }
              frame 16 {
                # "SOH过低"
                n3139 = disable-structure shown="启用" {
                  disable-tunnel: [w8138 w8146] -> w8125
                  disable-tunnel: w8124 -> [w8135 _]
                  disable-tunnel: [w8127 w8146] -> w8123
                  frame Disabled {
                    n3140 = Unbundle By Name(w8135) -> ("SOH过低"=w8134:dbl)
                    n3141 = call "输入分辨率计算-EV05.vi"("1字节?"=FALSE, "数值"=w8134, "偏移量"=0.0, "分辨率"=0.1) -> ("低字节"=w8136:dbl, "高字节1"=w8137:dbl)  [unwired: 1 in, 5 out]
                    n3142 = call "二进制解析-8.6.vi"("索引"=4, "数值"=w8137) -> ("低位子数组"=w8140:i32[])  [unwired: 3 out]
                    n3143 = call "二进制解析-8.6.vi"("索引"=4, "数值"=w8136) -> ("低位子数组"=w8129:i32[], "高位子数组"=w8139:i32[])  [unwired: 2 out]
                    n3144 = call "二进制解析-8.6.vi"("索引"=4, "数值"=0) -> ("低位子数组"=w8130:i32[])  [unwired: 3 out]
                    n3145 = Insert Into Array(array=w8140, new element=w8139) -> (w8133:i32[])  [unwired: 1 in]
                    n3146 = Insert Into Array(array=w8129, new element=w8130) -> (w8128:i32[])  [unwired: 1 in]
                    n3147 = call "数值二进制转十进制-8.6.vi"("子数组"=w8133) -> ("十进制数值"=w8138:i32)  [unwired: 4 out]
                    n3148 = call "数值二进制转十进制-8.6.vi"("子数组"=w8128) -> ("十进制数值"=w8127:i32)  [unwired: 4 out]
                  }
                  frame Enabled {
                    w8146 = 255 ("高字节1")
                  }
                }
                n3149 = Build Array(w8125, w8123) -> (w8126:i32[])
              }
            }
            n3150 = Insert Into Array(array=w7931, new element=w7932) -> (w7930:dbl[])  [unwired: 1 in]
          }
          n3151 = Build Array(w7927) -> (w7926:dbl[][])
          n3152 = Build Array("一级故障阀值") -> (w7917:string[])
        }
        frame "放电电流过高(2)" {
          n3153 = Unbundle By Name(w8152) -> ("一级故障 2"=w8153:refnum<vi>)
          n3154 = property class="Clust (严格)"(reference=w8153) -> ("Value"=w8151:T4)  [unwired: 1 in, 2 out]
          n3155 = for {
            N: 17 -> [_]
            tunnel: w8151 -> [w8163]
            shift-right: [w8160] -> w8157
            shift-left: dbl[] [] -> [w8161]
            i -> [w8164]
            n3156 = case shown="12" w8164 {
              tunnel: w8163 -> [w8165 w8176 w8187 w8197 w8207 w8217 w8229 w8241 w8253 w8265 w8277 w8289 w8303 w8324 w8336 w8345 w8354]
              tunnel: [w8166 w8177 w8188 w8198 w8208 w8219 w8231 w8243 w8255 w8267 w8279 w8290 w8312 w8327 w8335 w8344 w8356] -> w8162
              frame 0, Default {
                # "总电压过高"
                n3157 = disable-structure shown="启用" {
                  disable-tunnel: [w8172 w8175] -> w8168
                  disable-tunnel: [w8171 w8175] -> w8167
                  disable-tunnel: w8165 -> [w8170 _]
                  frame Disabled {
                    n3158 = Unbundle By Name(w8170) -> ("总电压过高"=w8169:dbl)
                    n3159 = call "输入分辨率计算-EV05.vi"("1字节?"=FALSE, "数值"=w8169, "分辨率"=0.1) -> ("低字节"=w8172:dbl, "高字节1"=w8171:dbl)  [unwired: 2 in, 5 out]
                  }
                  frame Enabled {
                    w8175 = 255 ("高字节1")
                  }
                }
                n3160 = Build Array(w8167, w8168) -> (w8166:i32[])
              }
              frame 1 {
                # "总电压过低"
                n3161 = disable-structure shown="启用" {
                  disable-tunnel: [w8183 w8186] -> w8179
                  disable-tunnel: [w8182 w8186] -> w8178
                  disable-tunnel: w8176 -> [w8181 _]
                  frame Disabled {
                    n3162 = Unbundle By Name(w8181) -> ("总电压过低"=w8180:dbl)
                    n3163 = call "输入分辨率计算-EV05.vi"("1字节?"=FALSE, "数值"=w8180, "分辨率"=0.1) -> ("低字节"=w8183:dbl, "高字节1"=w8182:dbl)  [unwired: 2 in, 5 out]
                  }
                  frame Enabled {
                    w8186 = 255 ("高字节1")
                  }
                }
                n3164 = Build Array(w8178, w8179) -> (w8177:i32[])
              }
              frame 2 {
                # "温度过高"
                n3165 = disable-structure shown="启用" {
                  disable-tunnel: [w8193 255 ("高字节1")] -> w8189
                  disable-tunnel: w8187 -> [w8191 _]
                  frame Disabled {
                    n3166 = Unbundle By Name(w8191) -> ("温度过高"=w8190:dbl)
                    n3167 = call "输入分辨率计算-EV05.vi"("1字节?"=TRUE, "数值"=w8190, "偏移量"=-40.0, "分辨率"=1.0) -> ("高字节1"=w8193:dbl)  [unwired: 1 in, 6 out]
                  }
                  frame Enabled {
                  }
                }
                n3168 = Build Array(w8189) -> (w8188:i32[])
              }
              frame 3 {
                # "温度过低"
                n3169 = disable-structure shown="启用" {
                  disable-tunnel: [w8203 255 ("高字节1")] -> w8199
                  disable-tunnel: w8197 -> [w8201 _]
                  frame Disabled {
                    n3170 = Unbundle By Name(w8201) -> ("温度过低"=w8200:dbl)
                    n3171 = call "输入分辨率计算-EV05.vi"("1字节?"=TRUE, "数值"=w8200, "偏移量"=-40.0, "分辨率"=1.0) -> ("高字节1"=w8203:dbl)  [unwired: 1 in, 6 out]
                  }
                  frame Enabled {
                  }
                }
                n3172 = Build Array(w8199) -> (w8198:i32[])
              }
              frame 4 {
                # "整组温度不均衡"
                n3173 = disable-structure shown="启用" {
                  disable-tunnel: [w8213 255 ("高字节1")] -> w8209
                  disable-tunnel: w8207 -> [w8211 _]
                  frame Disabled {
                    n3174 = Unbundle By Name(w8211) -> ("整组温度不均衡"=w8210:dbl)
                    n3175 = call "输入分辨率计算-EV05.vi"("1字节?"=TRUE, "数值"=w8210, "偏移量"=0.0, "分辨率"=1.0) -> ("高字节1"=w8213:dbl)  [unwired: 1 in, 6 out]
                  }
                  frame Enabled {
                  }
                }
                n3176 = Build Array(w8209) -> (w8208:i32[])
              }
              frame 5 {
                # "单组电压不均衡"
                n3177 = disable-structure shown="启用" {
                  disable-tunnel: [w8225 w8228] -> w8220
                  disable-tunnel: [w8223 w8228] -> w8218
                  disable-tunnel: w8217 -> [w8222 _]
                  frame Disabled {
                    n3178 = Unbundle By Name(w8222) -> ("单组电压不均衡"=w8221:dbl)
                    n3179 = call "输入分辨率计算-EV05.vi"("1字节?"=FALSE, "数值"=w8221, "偏移量"=0.0, "分辨率"=0.001) -> ("低字节"=w8223:dbl, "高字节1"=w8225:dbl)  [unwired: 1 in, 5 out]
                  }
                  frame Enabled {
                    w8228 = 255 ("高字节1")
                  }
                }
                n3180 = Build Array(w8220, w8218) -> (w8219:i32[])
              }
              frame 6 {
                # "整组电压不均衡"
                n3181 = disable-structure shown="启用" {
                  disable-tunnel: [w8237 w8240] -> w8232
                  disable-tunnel: [w8235 w8240] -> w8230
                  disable-tunnel: w8229 -> [w8234 _]
                  frame Disabled {
                    n3182 = Unbundle By Name(w8234) -> ("整组电压不均衡"=w8233:dbl)
                    n3183 = call "输入分辨率计算-EV05.vi"("1字节?"=FALSE, "数值"=w8233, "偏移量"=0.0, "分辨率"=0.001) -> ("低字节"=w8235:dbl, "高字节1"=w8237:dbl)  [unwired: 1 in, 5 out]
                  }
                  frame Enabled {
                    w8240 = 255 ("高字节1")
                  }
                }
                n3184 = Build Array(w8232, w8230) -> (w8231:i32[])
              }
              frame 7 {
                # "单体电压过高"
                n3185 = disable-structure shown="启用" {
                  disable-tunnel: [w8249 w8252] -> w8244
                  disable-tunnel: [w8247 w8252] -> w8242
                  disable-tunnel: w8241 -> [w8246 _]
                  frame Disabled {
                    n3186 = Unbundle By Name(w8246) -> ("单体电压过高"=w8245:dbl)
                    n3187 = call "输入分辨率计算-EV05.vi"("1字节?"=FALSE, "数值"=w8245, "偏移量"=0.0, "分辨率"=0.001) -> ("低字节"=w8247:dbl, "高字节1"=w8249:dbl)  [unwired: 1 in, 5 out]
                  }
                  frame Enabled {
                    w8252 = 255 ("高字节1")
                  }
                }
                n3188 = Build Array(w8244, w8242) -> (w8243:i32[])
              }
              frame 8 {
                # "单体电压过低"
                n3189 = disable-structure shown="启用" {
                  disable-tunnel: [w8261 w8264] -> w8256
                  disable-tunnel: [w8259 w8264] -> w8254
                  disable-tunnel: w8253 -> [w8258 _]
                  frame Disabled {
                    n3190 = Unbundle By Name(w8258) -> ("单体电压过低"=w8257:dbl)
                    n3191 = call "输入分辨率计算-EV05.vi"("1字节?"=FALSE, "数值"=w8257, "偏移量"=0.0, "分辨率"=0.001) -> ("低字节"=w8259:dbl, "高字节1"=w8261:dbl)  [unwired: 1 in, 5 out]
                  }
                  frame Enabled {
                    w8264 = 255 ("高字节1")
                  }
                }
                n3192 = Build Array(w8256, w8254) -> (w8255:i32[])
              }
              frame 9 {
                # "充电电流过高"
                n3193 = disable-structure shown="启用" {
                  disable-tunnel: [w8273 w8276] -> w8268
                  disable-tunnel: [w8271 w8276] -> w8266
                  disable-tunnel: w8265 -> [w8270 _]
                  frame Disabled {
                    n3194 = Unbundle By Name(w8270) -> ("充电电流过高"=w8269:dbl)
                    n3195 = call "输入分辨率计算-EV05.vi"("1字节?"=FALSE, "数值"=w8269, "偏移量"=-3000.0, "分辨率"=0.1) -> ("低字节"=w8271:dbl, "高字节1"=w8273:dbl)  [unwired: 1 in, 5 out]
                  }
                  frame Enabled {
                    w8276 = 255 ("高字节1")
                  }
                }
                n3196 = Build Array(w8268, w8266) -> (w8267:i32[])
              }
              frame 10 {
                # "放电电流过高"
                n3197 = disable-structure shown="启用" {
                  disable-tunnel: [w8285 w8288] -> w8280
                  disable-tunnel: [w8283 w8288] -> w8278
                  disable-tunnel: w8277 -> [w8282 _]
                  frame Enabled {
                    n3198 = Unbundle By Name(w8282) -> ("放电电流过高"=w8281:dbl)
                    n3199 = call "输入分辨率计算-EV05.vi"("1字节?"=FALSE, "数值"=w8281, "偏移量"=0.0, "分辨率"=0.1) -> ("低字节"=w8283:dbl, "高字节1"=w8285:dbl)  [unwired: 1 in, 5 out]
                  }
                  frame Disabled {
                    w8288 = 255 ("高字节1")
                  }
                }
                n3200 = Build Array(w8280, w8278) -> (w8279:dbl[])
              }
              frame 11 {
                # "单组温度不均衡"
                n3201 = disable-structure shown="启用" {
